vi "Queue New Launcher Command.vi"(8 "error in (no error)":errorcluster, 10 "New Launcher":T1, 11 "CIFPluginManager in":refnum<class "CIFPluginManager.lvclass">) -> (0 "error out":errorcluster)   [LabVIEW 2021, in "CIFPluginManager.lvclass"]
uses:
  CIFPluginManager.lvclass
  CIFPluginManager.lvclass/CIFPluginManager.ctl
  typedef/Loader Type.ctl
  typedef/Loader Load Info.ctl
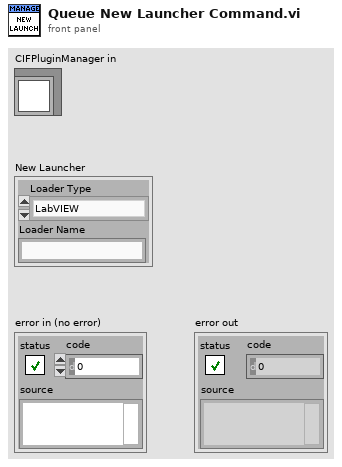
[diagram p1: front panel]
types:
  T1 = typedef "CIFPluginManager.lvclass/Loader Load Info.ctl" = cluster{"Loader Type":T2, "Loader Name":string}
  T2 = typedef "CIFPluginManager.lvclass/Loader Type.ctl" = enum16{"LabVIEW"}
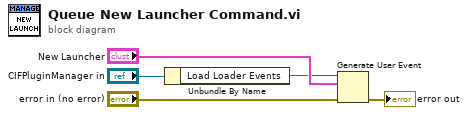
[diagram p0: block diagram]
diagram:
  n1 = Unbundle By Name("CIFPluginManager in") -> ("Load Loader Events"=w1:refnum<user-event>)
  n2 = Generate User Event(user event=w1, event data cluster="New Launcher", error in="error in (no error)") -> (error out=→"error out":errorcluster)  [unwired: 1 in, 1 out]
